vi "Init Komponentenauswahl.vi"(8 "Fehler (Eingang, kein Fehler)":errorcluster, 9 "Kontroll-Interferent: (Eingang)":refnum<vi>, 10 "Refernz-Interferent: (Eingang)":refnum<vi>, 11 "Komponente: (Eingang)":refnum<vi>) -> (0 "Fehler (Ausgang)":errorcluster, 1 "Kontroll-Interferent: (Ausgang)":refnum<vi>, 2 "Refernz-Interferent:  (Ausgang)":refnum<vi>, 3 "Komponente: (Ausgang)":refnum<vi>, 5 "Komponenten":T1)   [LabVIEW 2020, in "EPA 1065.lvlib" / "HovaCAL Interference verificaton.lvlib"]
uses:
  HovaCAL Interference verificaton.lvlib
  Komponenten.ctl
  Visualisierungs Elemente/String - Ausgabefeld.ctl
  Seiten/FT-IR/FGV FT-IR Gasliste Aktionen.ctl
  Aktion Index uebersetzten.ctl
  Seiten/FT-IR/FT-IR.lvlib
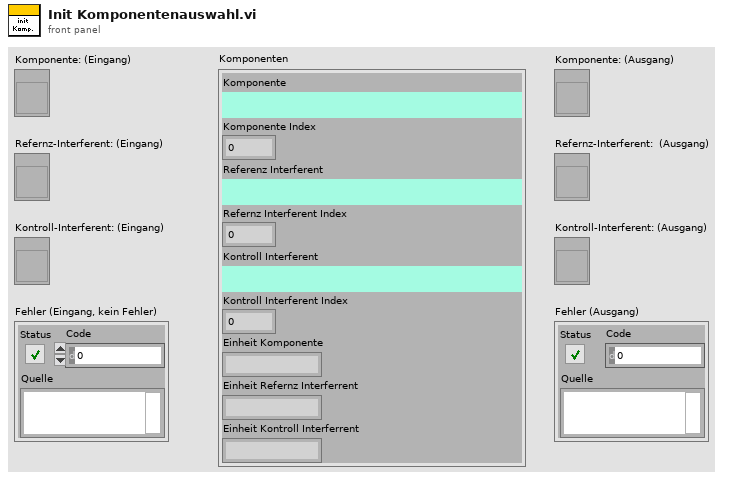
[diagram p1: front panel]
types:
  T1 = typedef "EPA 1065.lvlib/HovaCAL Interference verificaton.lvlib/Komponenten.ctl" = cluster{"Komponente":T2, "Komponente Index":i32, "Referenz Interferent":T2, "Refernz Interferent Index":i32, "Kontroll Interferent":T2, "Kontroll Interferent Index":i32, "Einheit Komponente":string, "Einheit Refernz Interferrent":string, "Einheit Kontroll Interferrent":string}
  T2 = typedef "String - Ausgabefeld.ctl" = string
  T3 = typedef "EPA 1065.lvlib/HovaCAL Interference verificaton.lvlib/Aktion Index uebersetzten.ctl" = enum16{"lesen", "schreiben", "auswerten", "Referenzwert"}
  T4 = typedef "FT-IR.lvlib/FGV FT-IR Gasliste Aktionen.ctl" = enum16{"lesen", "Gasliste FT-IR", "Gasliste ausgelesen", "laden", "speichern", "löschen"}
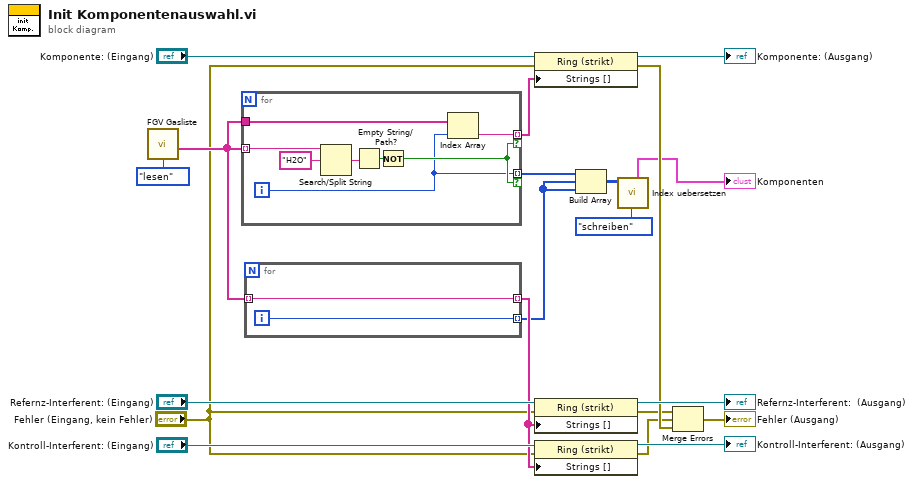
[diagram p0: block diagram]
diagram:
  n1 = call "FGV Gasliste.vi"("Aktionen"=FGV_FT-IR_Gasliste_Aktionen."lesen") -> ("Aktuelle Gasliste gesamt"=w5:T2[])  [unwired: 8 in, 2 out]
  n2 = for {
    tunnel: w5 -> [w23] mode=indexing
    tunnel: w5 -> [w22]
    tunnel: [w25] -> w11 mode=indexing if=w24
    tunnel: [w21] -> w16 mode=indexing if=w24
    i -> [w21]
    n3 = Search/Split String(string=w23, search string/char (-)="H2O" ("Such-String/-Zeichen (-)")) -> (match + rest of string=w27:T2)  [unwired: 1 in, 2 out]
    n4 = Empty String/Path?(string/path=w27) -> (empty?=w28:bool)
    n5 = Not(x=w28) -> (.not. x?=w24:bool)
    n6 = Index Array(array=w22, index=w21) -> (element=w25:T2)
  }
  n7 = for {
    tunnel: [w30] -> w4 mode=indexing
    tunnel: w5 -> [w30] mode=indexing
    tunnel: [w29] -> w2 mode=indexing
    i -> [w29]
  }
  n8 = property class="Ring (strikt)"(reference="Komponente: (Eingang)", error in="Fehler (Eingang, kein Fehler)", "Strings []"=w11) -> (reference out=→"Komponente: (Ausgang)":refnum<vi>, error out=w17:errorcluster)
  n9 = property class="Ring (strikt)"(reference="Refernz-Interferent: (Eingang)", error in="Fehler (Eingang, kein Fehler)", "Strings []"=w4) -> (reference out=→"Refernz-Interferent:  (Ausgang)":refnum<vi>, error out=w13:errorcluster)
  n10 = property class="Ring (strikt)"(reference="Kontroll-Interferent: (Eingang)", error in="Fehler (Eingang, kein Fehler)", "Strings []"=w4) -> (reference out=→"Kontroll-Interferent: (Ausgang)":refnum<vi>, error out=w15:errorcluster)
  n11 = Build Array(w16, w2, w2) -> (w6:i32[][])
  n12 = call "Index uebersetzen.vi"("Aktion"=Aktion_Index_uebersetzten."schreiben", "Index Array in"=w6) -> ("Komponenten"=→"Komponenten":T1)  [unwired: 5 in, 4 out]
  n13 = Merge Errors(w13, w15, w17) -> (→"Fehler (Ausgang)":errorcluster)
